vi "Get Chart Area.vi"(9 "Draw Area Size":T1) -> (1 "Chart Area Size":cluster{"Width":dbl, "Height":dbl}, 3 "Height":dbl)   [LabVIEW 2016, in "CML UI.lvlib" / "Circular Cue Helper.lvlib"]
doc: "Get Chart Area from the Draw Area Size. In this example, the height and width are both equal to Height in Draw Area Size/2."
uses:
  <vilib>/Utility/miscctls.llb/LVBoundsTypeDef.ctl
  Circular Cue Helper.lvlib
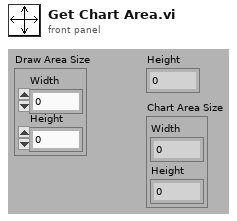
[diagram p1: front panel]
types:
  T1 = typedef "LVBoundsTypeDef.ctl" = cluster{"Width":u32, "Height":u32}
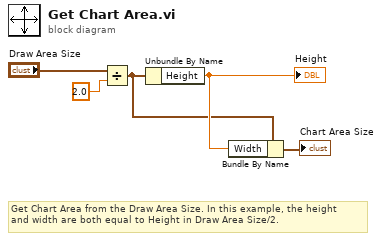
[diagram p0: block diagram]
diagram:
  # "Get Chart Area from the Draw Area Size. In this example, the height \nand width are both equal to Height in Draw Area Size/2."
  n1 = Divide(x="Draw Area Size", y=2.0) -> (x/y=w3:cluster{"Width":dbl, "Height":dbl})
  n2 = Unbundle By Name(w3) -> ("Height"=w4:dbl)
  "Height" <- w4
  n3 = Bundle By Name(cluster=w3, "Width"=w4) -> (→"Chart Area Size":cluster{"Width":dbl, "Height":dbl})
